vi "Create HTML.vi"(7 "FP Reference":refnum<class "Web Front Panel.lvclass">, 8 "error in (no error)":errorcluster, 9 "Panel Origin":T1, 10 "VI Name":string, 11 "Boolean In":refnum<class "Boolean.lvclass">) -> (0 "error out":errorcluster, 1 "js code for controls":string, 2 "js variables":string, 3 "Boolean Out":refnum<class "Boolean.lvclass">, 4 "script dependencies":string[](array[string]), 5 "HTML":string, 6 "js code for indicators":string)   [LabVIEW 2015, in "Front Panel Publisher.lvlib" / "Boolean.lvclass"]
uses:
  Boolean.lvclass
  Web Front Panel_class/Web Front Panel.lvclass
  <vilib>/Utility/miscctls.llb/LVPointTypeDef.ctl
  Text_class/Text.lvclass
  Object_class/Object.lvclass
  Control_class/Control.lvclass
  Front Panel Publisher.lvlib
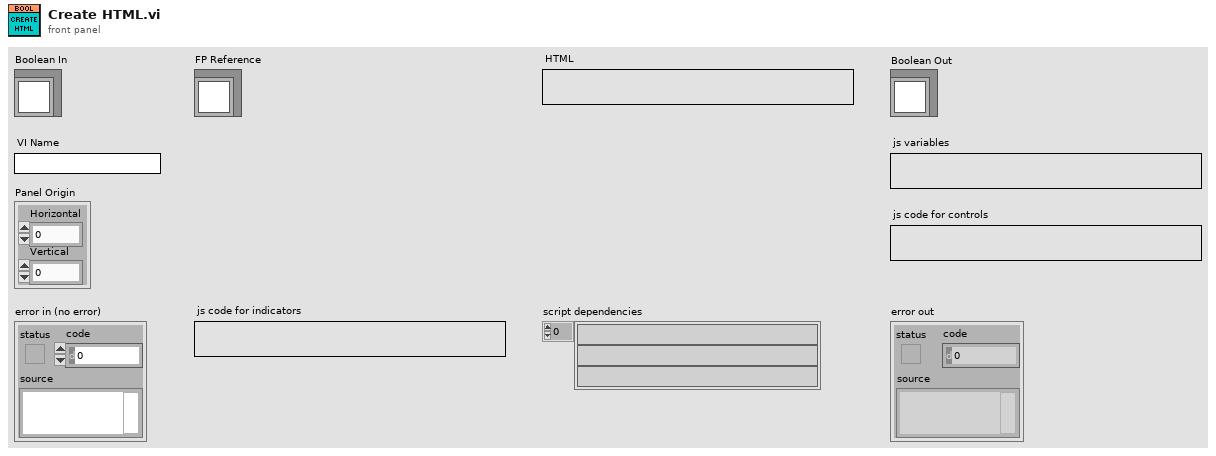
[diagram p1: front panel]
types:
  T1 = typedef "LVPointTypeDef.ctl" = cluster{"Horizontal":i16, "Vertical":i16}
  T2 = typedef "Front Panel Publisher.lvlib/Object.lvclass/Attributes.ctl" = cluster{"UID":i32, "Type":string, "Coordinates":T3, "Reference":refnum<vi>}
  T3 = typedef "Front Panel Publisher.lvlib/Object.lvclass/Coordinates.ctl" = cluster{"Left":i32, "Top":i32, "Height":u32, "Width":u32}
  T4 = typedef "Front Panel Publisher.lvlib/Control.lvclass/Attributes.ctl" = cluster{"Description":string, "Indicator":bool, "Default Value":variant, "Control Index":i32, "Label":refnum<class "Text.lvclass">, "Caption":refnum<class "Text.lvclass">, "Image b64":string, "Use Picture":bool, "Value Only":bool}
  T5 = typedef "Front Panel Publisher.lvlib/Boolean.lvclass/Attributes.ctl" = cluster{"Boolean ref":refnum<vi>, "Switching":bool, "Boolean Strings":string[], "Text":refnum<class "Text.lvclass">, "Images b64":string[]}
  T6 = typedef "LVRectTypeDef.ctl" = cluster{"Left":i16, "Top":i16, "Right":i16, "Bottom":i16}
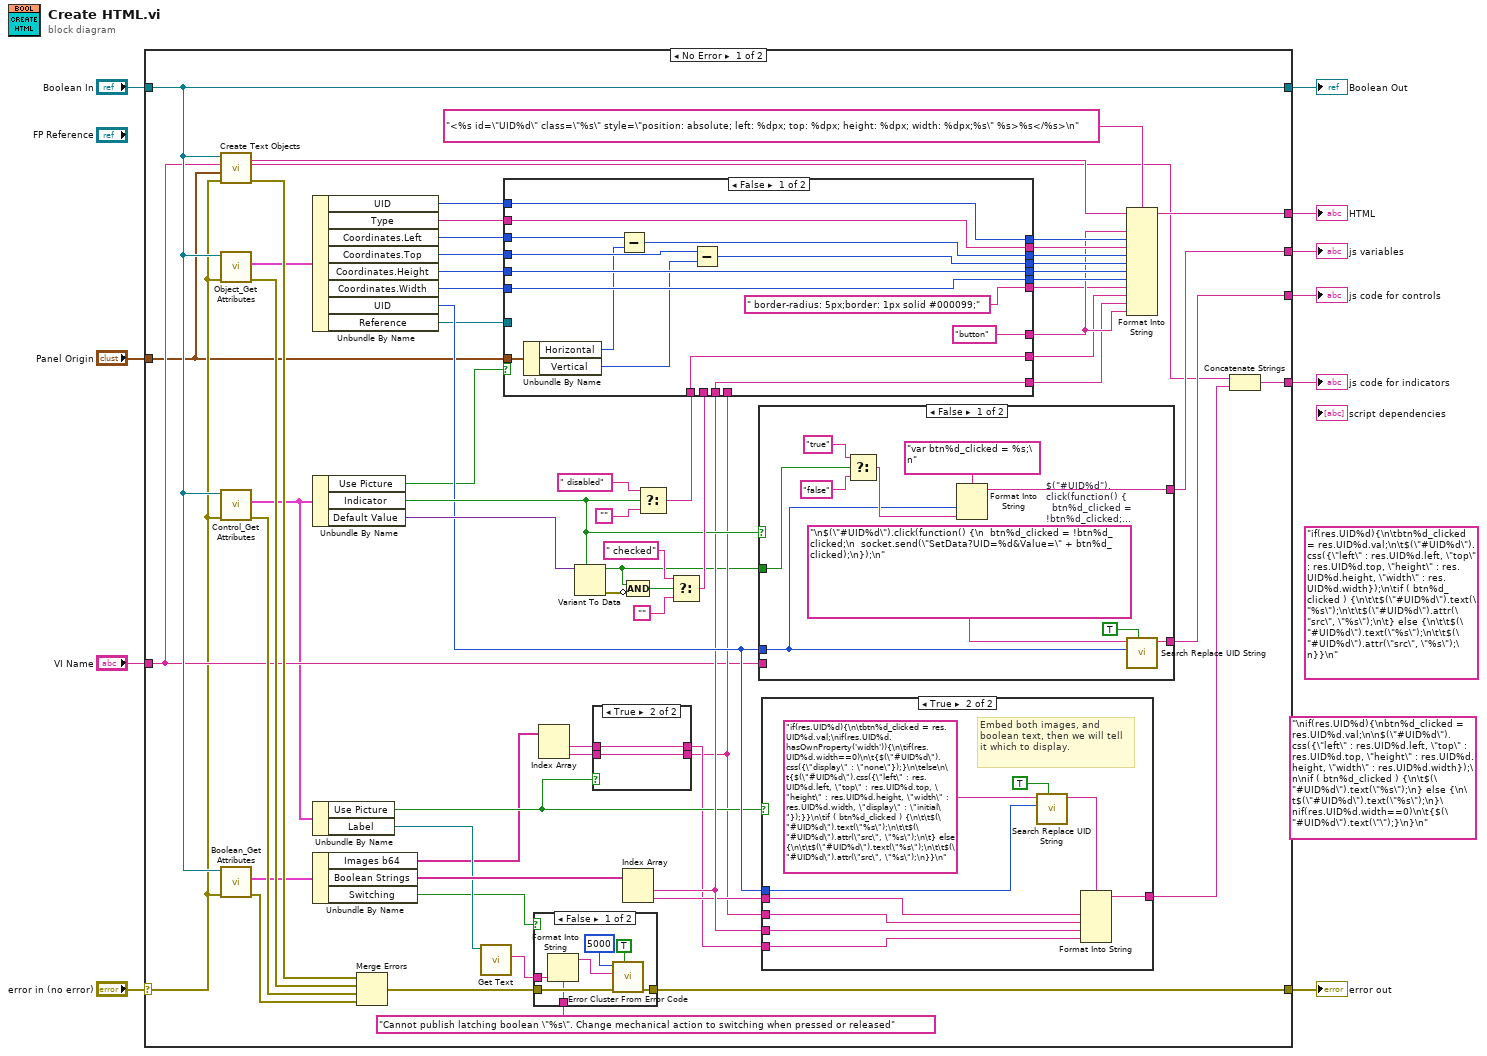
[diagram p0: block diagram]
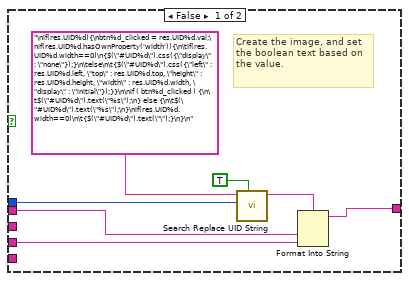
[diagram p2: hidden frame]
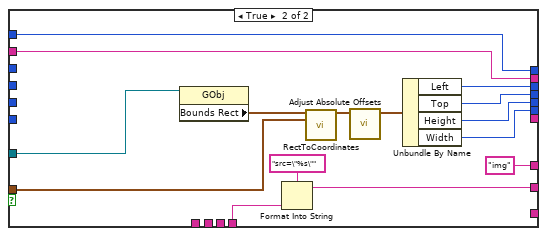
[diagram p6: hidden frame]
diagram:
  (unwired) "if(res.UID%d){\n\tbtn%d_clicked = res.UID%d.val;\n\t$(\"#UID%d\").css({\"left\" : res.UID%d.left, \"top\" : res.UID%d.top, \"height\" : res.UID%d.height, \"width\" : res.UID%d.width});\n\tif ( btn%d_clicked ) {\n\t\t$(\"#UID%d\").text(\"%s\");\n\t\t$(\"#UID%d\").attr(\"src\", \"%s\");\n\t} else {\n\t\t$(\"#UID%d\").text(\"%s\");\n\t\t$(\"#UID%d\").attr(\"src\", \"%s\");\n}}\n"
  (unwired) "\nif(res.UID%d){\nbtn%d_clicked = res.UID%d.val;\n\n$(\"#UID%d\").css({\"left\" : res.UID%d.left, \"top\" : res.UID%d.top, \"height\" : res.UID%d.height, \"width\" : res.UID%d.width});\n\nif ( btn%d_clicked ) {\n\t$(\"#UID%d\").text(\"%s\");\n} else {\n\t$(\"#UID%d\").text(\"%s\");\n}\nif(res.UID%d.width==0)\n\t{$(\"#UID%d\").text(\"\");}\n}\n"
  n1 = case shown="No Error" "error in (no error)" {
    selector: "error in (no error)" -> [w20 w142]
    tunnel: [w21 w142] -> w9
    tunnel: [w24 w141] -> w7
    tunnel: "Boolean In" -> [w24 w141]
    tunnel: [w67 _] -> w6
    tunnel: [w42 _] -> w5
    tunnel: [w41 _] -> w4
    tunnel: [w16 _] -> w3
    tunnel: "VI Name" -> [w23 _]
    tunnel: "Panel Origin" -> [w11 _]
    frame No Error {
      n2 = call-dynamic "Create Text Objects.vi"("error in (no error)"=w20, "Panel Origin"=w11, "VI Name"=w23, "Control In"=w24) -> ("error out"=w69:errorcluster, "JS Indicator"=w13:string, "HTML"=w22:string)  [unwired: 4 in, 1 out]
      n3 = call "Object_Get Attributes.vi"("error in (no error)"=w20, "Object In"=w24) -> ("error out"=w70:errorcluster, "Data"=w66:T2)  [unwired: 6 in, 2 out]
      n4 = call "Control_Get Attributes.vi"("error in (no error)"=w20, "Control In"=w24) -> ("error out"=w71:errorcluster, "Data"=w19:T4)  [unwired: 6 in, 2 out]
      n5 = call "Boolean_Get Attributes.vi"("error in (no error)"=w20, "Boolean In"=w24) -> ("error out"=w73:errorcluster, "Data"=w53:T5)  [unwired: 6 in, 2 out]
      n6 = Unbundle By Name(w66) -> ("UID"=w65:i32, "Type"=w64:string, "Coordinates.Left"=w63:i32, "Coordinates.Top"=w62:i32, "Coordinates.Height"=w61:u32, "Coordinates.Width"=w60:u32, "UID"=w38:i32, "Reference"=w14:refnum<vi>)
      n7 = Unbundle By Name(w19) -> ("Use Picture"=w35:bool, "Indicator"=w43:bool, "Default Value"=w46:variant)
      n8 = Unbundle By Name(w19) -> ("Use Picture"=w32:bool, "Label"=w28:refnum<class "Text.lvclass">)
      n9 = Unbundle By Name(w53) -> ("Images b64"=w12:string[], "Boolean Strings"=w44:string[], "Switching"=w25:bool)
      n10 = Merge Errors(w69, w70, w71, w73) -> (w72:errorcluster)
      n11 = call-dynamic "Get Text.vi"("Text In"=w28) -> ("Text"=w27:string)  [unwired: 8 in, 2 out]
      n12 = case shown="False" w25 {
        tunnel: [w97 w98] -> w21
        tunnel: w72 -> [w96 w98]
        tunnel: w27 -> [w93 _]
        tunnel: "Cannot publish latching boolean \"%s\". Change mechanical action to switching when pressed or released" -> [w92 _]
        frame False {
          n13 = Format Into String(format string=w92, w93) -> (resulting string=w91:string)  [unwired: 2 in, 1 out]
          n14 = call <vilib>:"Error Cluster From Error Code.vi"("show call chain? (False)"=TRUE, "error in (no error)"=w96, "error message (\"\")"=w91, "error code (0)"=5000) -> ("error out"=w97:errorcluster)  [unwired: 5 in]
        }
        frame True {
        }
      }
      n15 = Index Array(array=w12) -> (element #1=w18:string, element #2=w17:string)  [unwired: 2 in]
      n16 = Variant To Data(type=w43, Variant=w46) -> (data=w29:bool, error out=w74:errorcluster)  [unwired: 1 in]
      n17 = case shown="True" w32 {
        tunnel: [_ w100] -> w30
        tunnel: [_ w99] -> w31
        tunnel: w17 -> [_ w100]
        tunnel: w18 -> [_ w99]
        frame False {
        }
        frame True {
        }
      }
      n18 = Index Array(array=w44) -> (element #1=w37:string, element #2=w36:string)  [unwired: 2 in]
      n19 = Compound Arithmetic op=AND(w29, invert w74) -> (w49:bool)
      n20 = Select(t=" disabled", s=w43, f="") -> (s? t:f=w50:string)
      n21 = Select(t=" checked", s=w49, f="") -> (s? t:f=w45:string)
      n22 = case shown="False" w35 {
        tunnel: ["button" "img"] -> w40
        tunnel: w50 -> [w116 _]
        tunnel: w45 -> [_ _]
        tunnel: [w124 _] -> w39
        tunnel: w37 -> [w124 _]
        tunnel: [w116 w135] -> w33
        tunnel: [w122 w139] -> w58
        tunnel: w64 -> [w122 w139]
        tunnel: [w123 w138] -> w59
        tunnel: w65 -> [w123 w138]
        tunnel: [w115 w134] -> w57
        tunnel: w63 -> [w121 _]
        tunnel: [w114 w133] -> w56
        tunnel: w62 -> [w120 _]
        tunnel: [w118 w131] -> w54
        tunnel: w60 -> [w118 _]
        tunnel: w61 -> [w119 _]
        tunnel: [w119 w132] -> w55
        tunnel: [" border-radius: 5px;border: 1px solid #000099;" _] -> w34
        tunnel: w30 -> [_ w136]
        tunnel: w14 -> [_ w130]
        tunnel: w11 -> [w113 w126]
        frame False {
          n23 = Unbundle By Name(w113) -> ("Horizontal"=w112:i16, "Vertical"=w111:i16)
          n24 = Subtract(x=w121, y=w112) -> (x-y=w115:i32)
          n25 = Subtract(x=w120, y=w111) -> (x-y=w114:i32)
        }
        frame True {
          n26 = property class="GObj"(reference=w130) -> ("Bounds Rect"=w128:T6)  [unwired: 1 in, 2 out]
          n27 = Format Into String(format string="src=\"%s\"", w136) -> (resulting string=w135:string)  [unwired: 2 in, 1 out]
          n28 = call "RectToCoordinates.vi"("Rect"=w128, "Panel Origin"=w126) -> ("Coordinates"=w129:T3)  [unwired: 13 in]
          n29 = call "Adjust Absolute Offsets.vi"("Coordinates in"=w129) -> ("Coordinates out"=w127:T3)  [unwired: 8 in, 2 out]
          n30 = Unbundle By Name(w127) -> ("Left"=w134:i32, "Top"=w133:i32, "Height"=w132:u32, "Width"=w131:u32)
        }
      }
      n31 = case shown="False" w43 {
        tunnel: [w102 _] -> w41
        tunnel: w38 -> [w103 _]
        tunnel: [w110 _] -> w42
        tunnel: w23 -> [_ _]
        tunnel: w29 -> [w108 _]
        frame False {
          w104 = "\n$(\"#UID%d\").click(function() {\n  btn%d_clicked = !btn%d_clicked;\n  socket.send(\"SetData?UID=%d&Value=\" + btn%d_clicked);\n});\n"  # $("#UID%d").click(function() {   btn%d_clicked = !btn%d_clicked;   socket.send("SetData?UID=%d&Value=" + btn%d_clicked); });
          n32 = Select(t="true", s=w108, f="false") -> (s? t:f=w105:string)
          n33 = Format Into String(format string="var btn%d_clicked = %s;\n", w103, w105) -> (resulting string=w110:string)  [unwired: 2 in, 1 out]
          n34 = call "Search Replace UID String.vi"("Replace All Numeric Inputs"=TRUE, "UID"=w103, "Input String"=w104) -> ("Output String"=w102:string)  [unwired: 8 in]
        }
        frame True {
        }
      }
      n35 = case shown="True" w32 {
        tunnel: w36 -> [w81 w89]
        tunnel: w38 -> [w78 w83]
        tunnel: [w79 w90] -> w15
        tunnel: w37 -> [w80 w87]
        tunnel: w30 -> [_ w88]
        tunnel: w31 -> [_ w86]
        frame False {
          # "Create the image, and set the boolean text based on the value."
          n36 = call "Search Replace UID String.vi"("Replace All Numeric Inputs"=TRUE, "UID"=w78, "Input String"="\nif(res.UID%d){\nbtn%d_clicked = res.UID%d.val;\nif(res.UID%d.hasOwnProperty('width')){\n\tif(res.UID%d.width==0)\n{$(\"#UID%d\").css({\"display\" : \"none\"});}\n\telse\n\t{$(\"#UID%d\").css({\"left\" : res.UID%d.left, \"top\" : res.UID%d.top, \"height\" : res.UID%d.height, \"width\" : res.UID%d.width, \"display\" : \"initial\"});}}\n\nif ( btn%d_clicked ) {\n\t$(\"#UID%d\").text(\"%s\");\n} else {\n\t$(\"#UID%d\").text(\"%s\");\n}\nif(res.UID%d.width==0)\n\t{$(\"#UID%d\").text(\"\");}\n}\n") -> ("Output String"=w75:string)  [unwired: 8 in]
          n37 = Format Into String(format string=w75, w81, w80) -> (resulting string=w79:string)  [unwired: 2 in, 1 out]
        }
        frame True {
          # "Embed both images, and boolean text, then we will tell it which to display."
          n38 = call "Search Replace UID String.vi"("Replace All Numeric Inputs"=TRUE, "UID"=w83, "Input String"="if(res.UID%d){\n\tbtn%d_clicked = res.UID%d.val;\nif(res.UID%d.hasOwnProperty('width')){\n\tif(res.UID%d.width==0)\n\t{$(\"#UID%d\").css({\"display\" : \"none\"});}\n\telse\n\t{$(\"#UID%d\").css({\"left\" : res.UID%d.left, \"top\" : res.UID%d.top, \"height\" : res.UID%d.height, \"width\" : res.UID%d.width, \"display\" : \"initial\"});}}\n\tif ( btn%d_clicked ) {\n\t\t$(\"#UID%d\").text(\"%s\");\n\t\t$(\"#UID%d\").attr(\"src\", \"%s\");\n\t} else {\n\t\t$(\"#UID%d\").text(\"%s\");\n\t\t$(\"#UID%d\").attr(\"src\", \"%s\");\n}}\n") -> ("Output String"=w82:string)  [unwired: 8 in]
          n39 = Format Into String(format string=w82, w89, w88, w87, w86) -> (resulting string=w90:string)  [unwired: 2 in, 1 out]
        }
      }
      n40 = Format Into String(format string="<%s id=\"UID%d\" class=\"%s\" style=\"position: absolute; left: %dpx; top: %dpx; height: %dpx; width: %dpx;%s\" %s>%s</%s>\n", initial string=w22, w40, w59, w58, w57, w56, w55, w54, w34, w33, w39, w40) -> (resulting string=w67:string)  [unwired: 1 in, 1 out]
      n41 = Concatenate Strings(w13, w15) -> (w16:string)
    }
    frame Error {
    }
  }
  "error out" <- w9
  "Boolean Out" <- w7
  "HTML" <- w6
  "js variables" <- w5
  "js code for controls" <- w4
  "js code for indicators" <- w3
